vi "uLTV_main.vi"() -> ()   [LabVIEW 2021]
uses:
  <vilib>/myRIO/Instrument Drivers/Onboard IO/DIO/typedefs/DIO Reference.ctl
  <vilib>/myRIO/Common/Instrument Driver Framework/Utilities/typedefs/myRIO Generic Hardware Reference.ctl
  <vilib>/myRIO/Common/Instrument Driver Framework/Utilities/typedefs/Hardware Version Enum.ctl
  <vilib>/myRIO/Common/Instrument Driver Framework/Utilities/typedefs/myRIO v1.0 Reference.ctl
  <vilib>/myRIO/Common/Instrument Driver Framework/Utilities/typedefs/Generic FPGA Reference.ctl
  <vilib>/myRIO/Common/Instrument Driver Framework/myRIO v1.0/DIO/typedefs/DIO Channels List.ctl
  <vilib>/myRIO/Common/Instrument Driver Framework/myRIO v1.0/DIO/typedefs/DIO Channels Enum.ctl
  <vilib>/userDefined/High Color/nirio_resource_hc.ctl
  <vilib>/myRIO/Instrument Drivers/Onboard IO/PWM/typedefs/PWM Reference.ctl
  <vilib>/myRIO/Common/Instrument Driver Framework/myRIO v1.0/PWM/typedefs/PWM Channels Enum.ctl
  <vilib>/myRIO/Instrument Drivers/Onboard IO/PWM/typedefs/PWM Configuration.ctl
  <vilib>/myRIO/Common/Instrument Driver Framework/Utilities/vis/Is FPGA Ref Available.vi
  <vilib>/myRIO/Common/Instrument Driver Framework/myRIO v1.0/DIO/vis/myRIO v1.1 Open DIO.vi
  <vilib>/myRIO/Instrument Drivers/Onboard IO/DIO/vis/Write.vi
  <vilib>/myRIO/Common/Instrument Driver Framework/myRIO v1.0/PWM/vis/myRIO v1.1 Open PWM.vi
  <vilib>/myRIO/Instrument Drivers/Onboard IO/PWM/vis/Set Duty Cycle and Frequency.vi
  <vilib>/myRIO/Common/Instrument Driver Framework/Utilities/vis/Validate Channels.vi
  <vilib>/myRIO/Common/Instrument Driver Framework/myRIO v1.0/DIO/vis/myRIO v1.0 Reserve DIO.vi
  <vilib>/myRIO/Common/Instrument Driver Framework/myRIO v1.0/PWM/vis/myRIO v1.0 Reserve PWM.vi
  <vilib>/myRIO/Common/Instrument Driver Framework/myRIO v1.0/Resource Manager/vis/myRIO v1.0 Reserve Channel List.vi
  <vilib>/myRIO/Common/Instrument Driver Framework/myRIO v1.0/DIO/vis/myRIO v1.0 Build MUX Configuration DIO.vi
  <vilib>/myRIO/Common/Instrument Driver Framework/myRIO v1.0/PWM/vis/myRIO v1.0 Build MUX Configuration PWM.vi
  <vilib>/myRIO/Common/Instrument Driver Framework/myRIO v1.0/Resource Manager/vis/myRIO v1.0 Reserve Channel.vi
  <vilib>/myRIO/Common/Instrument Driver Framework/myRIO v1.0/Resource Manager/vis/myRIO v1.0 Unreserve Channel.vi
  <vilib>/myRIO/Common/Instrument Driver Framework/myRIO v1.0/Resource Manager/vis/myRIO v1.0 Create Configuration List.vi
  <vilib>/myRIO/Common/Instrument Driver Framework/myRIO v1.0/Resource Manager/vis/myRIO v1.0 Build Mutex Name.vi
  <vilib>/Utility/VariantDataType/GetNumericInfo.vi
  <vilib>/Utility/error.llb/Error Cluster From Error Code.vi
  <vilib>/myRIO/Common/Instrument Driver Framework/myRIO v1.0/myRIO v1.1 Open.vi
  <vilib>/myRIO/Common/Instrument Driver Framework/Utilities/vis/IO Manager.vi
  <vilib>/myRIO/Common/Instrument Driver Framework/Utilities/vis/Configuration Manager.vi
  <vilib>/myRIO/Common/Instrument Driver Framework/myRIO v1.0/Resource Manager/vis/myRIO v1.0 Configure IO.vi
  <vilib>/myRIO/Common/Instrument Driver Framework/myRIO v1.0/myRIO v1.0 Close.vi
  <vilib>/myRIO/Common/Instrument Driver Framework/myRIO v1.0/PWM/vis/myRIO v1.0 Write PWM.vi
  <vilib>/myRIO/Common/Instrument Driver Framework/myRIO v1.0/DIO/vis/myRIO v1.0 Write DIO.vi
  <vilib>/myRIO/Express VI/Onboard IO/PWM/PWM Express VI.xnode
  <vilib>/myRIO/Instrument Drivers/Onboard IO/PWM/vis/myRIO PWM Open.xnode
  <vilib>/myRIO/Express VI/Onboard IO/DO/DO Express VI.xnode
  <vilib>/myRIO/Instrument Drivers/Onboard IO/DIO/vis/myRIO DIO Open.xnode
  <vilib>/myRIO/Instrument Drivers/Onboard IO/PWM/PWM.lvlib
  <vilib>/myRIO/Instrument Drivers/Onboard IO/DIO/DIO.lvlib
panel:
  out "A/DIO0 (Pin 11) 4":bool
  out "A/DIO0 (Pin 11) 3":bool
  out "A/DIO0 (Pin 11) 2":bool
  out "A/DIO0 (Pin 11)":bool
  in  "Frequency [Hz]":dbl=1000.0
  out "Angle":dbl
  out "Magnitude":dbl
  in  "stop":bool
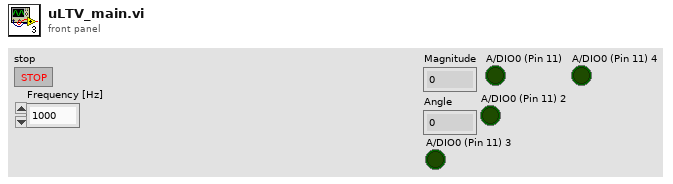
[diagram p1: front panel]
types:
  T1 = typedef "DIO.lvlib/DIO Reference.ctl" = cluster{"myRIO Reference":T2, "DIO Channels List":T6}
  T2 = typedef "myRIO Generic Hardware Reference.ctl" = cluster{"myRIO Model":T3, "myRIO Hardware Reference":T4}
  T3 = typedef "Hardware Version Enum.ctl" = enum16{"Unknown", "myRIO-1900", "myRIO-1950", "roboRIO", "NI ELVIS RIO CM", "ELVIS III"}
  T4 = typedef "myRIO v1.0 Reference.ctl" = cluster{"Generic FPGA Reference":T5, "Allow multiple opens":bool}
  T5 = typedef "Generic FPGA Reference.ctl" = refnum<k20>
  T6 = typedef "DIO Channels List.ctl" = T7[]
  T7 = typedef "DIO Channels Enum.ctl" = enum16{"Not Connected", "C/DIO0", "C/DIO1", "C/DIO2", "C/DIO3", "C/DIO4", "C/DIO5", "C/DIO6", "C/DIO7", "A/DIO0", "A/DIO1", "A/DIO2", "A/DIO3", "A/DIO4", "A/DIO5", "A/DIO6", "A/DIO7", "A/DIO8", "A/DIO9", "A/DIO10", "A/DIO11", "A/DIO12", "A/DIO13", "A/DIO14", "A/DIO15", "A/DIO16", "A/DIO17", "A/DIO18", "A/DIO19", "B/DIO0", "B/DIO1", "B/DIO2", "B/DIO3", "B/DIO4", "B/DIO5", "B/DIO6", "B/DIO7", "B/DIO8", "B/DIO9", "B/DIO10", "B/DIO11", "B/DIO12", "B/DIO13", "B/DIO14", "B/DIO15", "B/DIO16", "B/DIO17", "B/DIO18", "B/DIO19", "LED0", "LED1", "LED2", "LED3", "Button0", "DIO/DIO0", "DIO/DIO1", "DIO/DIO2", "DIO/DIO3", "DIO/DIO4", "DIO/DIO5", "DIO/DIO6", "DIO/DIO7", "DIO/DIO8", "DIO/DIO9", "SPI/CS0", "SPI/CS1", "SPI/CS2", "SPI/CS3", "LED RADIO (Green)", "LED RADIO (Red)", "LED COMM (Green)", "LED COMM (Red)", "LED MODE (Green)", "LED MODE (Red)"}
  T8 = typedef "nirio_resource_hc.ctl" = tag
  T9 = typedef "PWM.lvlib/PWM Reference.ctl" = cluster{"myRIO Reference":T2, "PWM Channels Enum":T10, "PWM Configuration":T11}
  T10 = typedef "PWM Channels Enum.ctl" = enum16{"Not Connected", "C/PWM0", "C/PWM1", "A/PWM0", "A/PWM1", "A/PWM2", "A/PWM3", "A/PWM4", "A/PWM5", "A/PWM6", "A/PWM7", "A/PWM8", "A/PWM9", "A/PWM10", "A/PWM11", "A/PWM12", "A/PWM13", "A/PWM14", "A/PWM15", "A/PWM16", "A/PWM17", "A/PWM18", "A/PWM19", "B/PWM0", "B/PWM1", "B/PWM2", "B/PWM3", "B/PWM4", "B/PWM5", "B/PWM6", "B/PWM7", "B/PWM8", "B/PWM9", "B/PWM10", "B/PWM11", "B/PWM12", "B/PWM13", "B/PWM14", "B/PWM15", "B/PWM16", "B/PWM17", "B/PWM18", "B/PWM19", "PWM/PWM0", "PWM/PWM1", "PWM/PWM2", "PWM/PWM3", "PWM/PWM4", "PWM/PWM5", "PWM/PWM6", "PWM/PWM7", "PWM/PWM8", "PWM/PWM9"}
  T11 = typedef "PWM.lvlib/PWM Configuration.ctl" = cluster{"Frequency":dbl, "Duty Cycle":dbl}
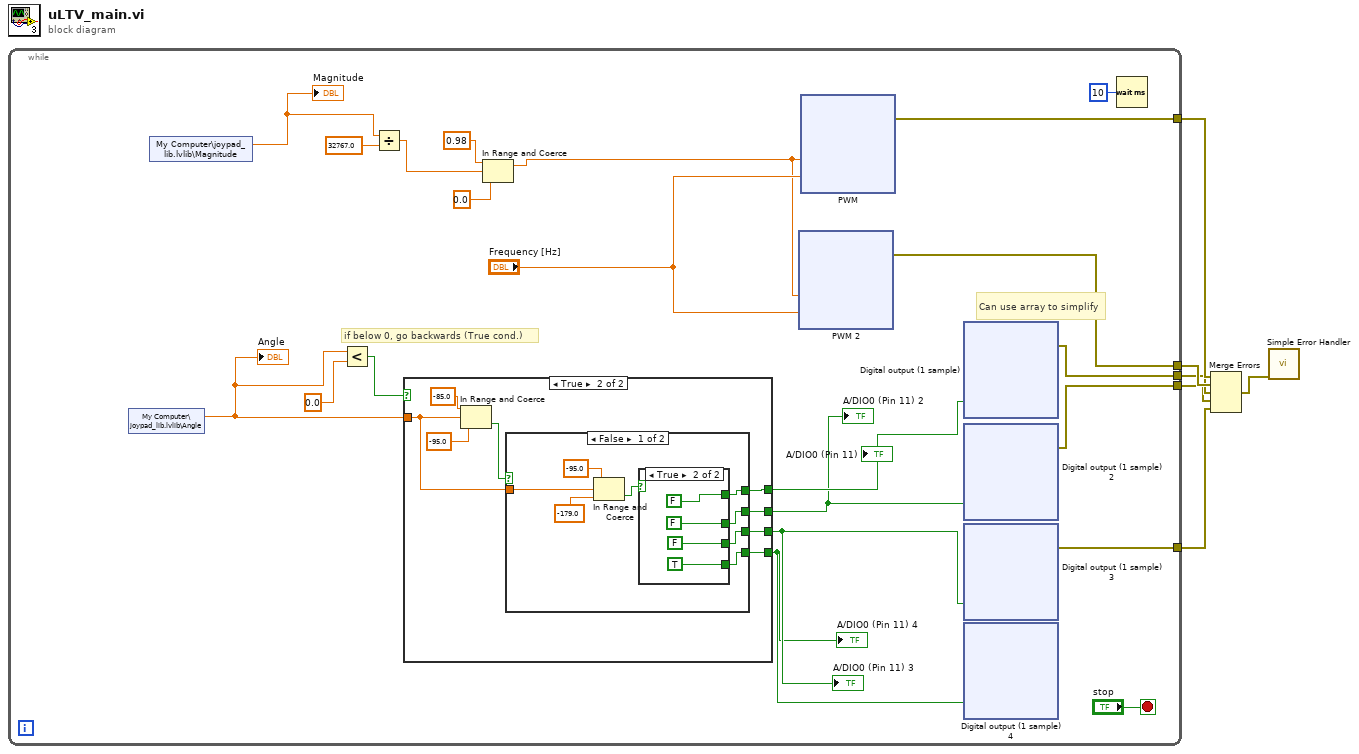
[diagram p0: block diagram]
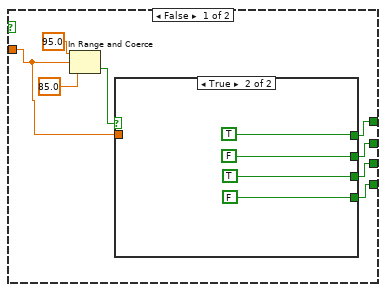
[diagram p2: hidden frame]
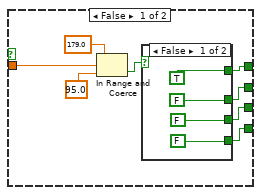
[diagram p3: hidden frame]
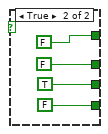
[diagram p4: hidden frame]
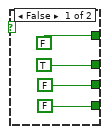
[diagram p5: hidden frame]
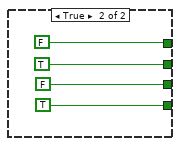
[diagram p6: hidden frame]
diagram:
  n1 = while {
    tunnel: [w17] -> w5
    tunnel: [w16] -> w4
    tunnel: [w15] -> w3
    tunnel: [w14] -> w2
    tunnel: [w13] -> w1
    stop <- "stop" stop-if-true
    # "Can use array to simplify"
    # "if below 0, go backwards (True cond.)"
    n2 = shared-variable "My Computer\\joypad_lib.lvlib\\Angle"() -> (w12:dbl)  [unwired: 1 in, 1 out]
    "Angle" <- w12
    n3 = shared-variable "My Computer\\joypad_lib.lvlib\\Magnitude"() -> (w22:dbl)  [unwired: 1 in, 1 out]
    "Magnitude" <- w22
    n4 = Less?(x=w12, y=0.0) -> (x < y?=w18:bool)
    n5 = Divide(x=w22, y=32767.0) -> (x/y=w21:dbl)
    n6 = case shown="True" w18 {
      tunnel: w12 -> [w172 w200]
      tunnel: [w171 w197] -> w11
      tunnel: [w170 w199] -> w9
      tunnel: [w169 w198] -> w8
      tunnel: [w168 w196] -> w7
      frame False {
        n7 = In Range and Coerce(upper limit=95.0, x=w172, lower limit=85.0) -> (In Range?=w173:bool)  [unwired: 1 out]
        n8 = case shown="True" w173 {
          tunnel: w172 -> [w181 _]
          tunnel: [w179 FALSE ("A/DIO0 (Pin 11)")] -> w170
          tunnel: [w178 TRUE ("A/DIO0 (Pin 11)")] -> w169
          tunnel: [w177 TRUE ("A/DIO0 (Pin 11)")] -> w171
          tunnel: [w176 FALSE ("A/DIO0 (Pin 11)")] -> w168
          frame False {
            n9 = In Range and Coerce(upper limit=179.0, x=w181, lower limit=95.0) -> (In Range?=w180:bool)  [unwired: 1 out]
            n10 = case shown="False" w180 {
              tunnel: [TRUE ("A/DIO0 (Pin 11)") FALSE ("A/DIO0 (Pin 11)")] -> w177
              tunnel: [FALSE ("A/DIO0 (Pin 11)") FALSE ("A/DIO0 (Pin 11)")] -> w179
              tunnel: [FALSE ("A/DIO0 (Pin 11)") TRUE ("A/DIO0 (Pin 11)")] -> w178
              tunnel: [FALSE ("A/DIO0 (Pin 11)") FALSE ("A/DIO0 (Pin 11)")] -> w176
              frame False {
              }
              frame True {
              }
            }
          }
          frame True {
          }
        }
      }
      frame True {
        n11 = In Range and Coerce(upper limit=-85.0, x=w200, lower limit=-95.0) -> (In Range?=w201:bool)  [unwired: 1 out]
        n12 = case shown="False" w201 {
          tunnel: w200 -> [w209 _]
          tunnel: [w207 TRUE ("A/DIO0 (Pin 11)")] -> w199
          tunnel: [w206 FALSE ("A/DIO0 (Pin 11)")] -> w198
          tunnel: [w205 FALSE ("A/DIO0 (Pin 11)")] -> w197
          tunnel: [w204 TRUE ("A/DIO0 (Pin 11)")] -> w196
          frame False {
            n13 = In Range and Coerce(upper limit=-95.0, x=w209, lower limit=-179.0) -> (In Range?=w208:bool)  [unwired: 1 out]
            n14 = case shown="True" w208 {
              tunnel: [FALSE ("A/DIO0 (Pin 11)") FALSE ("A/DIO0 (Pin 11)")] -> w205
              tunnel: [TRUE ("A/DIO0 (Pin 11)") FALSE ("A/DIO0 (Pin 11)")] -> w207
              tunnel: [FALSE ("A/DIO0 (Pin 11)") FALSE ("A/DIO0 (Pin 11)")] -> w206
              tunnel: [FALSE ("A/DIO0 (Pin 11)") TRUE ("A/DIO0 (Pin 11)")] -> w204
              frame False {
              }
              frame True {
              }
            }
          }
          frame True {
          }
        }
      }
    }
    "A/DIO0 (Pin 11)" <- w11
    "A/DIO0 (Pin 11) 2" <- w9
    "A/DIO0 (Pin 11) 3" <- w8
    "A/DIO0 (Pin 11) 4" <- w7
    n15 = In Range and Coerce(upper limit=0.98, x=w21, lower limit=0.0) -> (coerced(x)=w10:dbl)  [unwired: 1 out]
    n16 = xnode "PWM 2"("Duty Cycle"=w10, "Frequency [Hz]"="Frequency [Hz]") -> ("error out"=w16:errorcluster)  [unwired: 1 in]
    n17 = xnode "PWM"("Duty Cycle"=w10, "Frequency [Hz]"="Frequency [Hz]") -> ("error out"=w17:errorcluster)  [unwired: 1 in]
    n18 = xnode "Digital output (1 sample)"("A/DIO0 (Pin 11)"=w11) -> ("error out"=w15:errorcluster)  [unwired: 1 in]
    n19 = xnode "Digital output (1 sample) 2"("A/DIO1 (Pin 13)"=w9) -> ("error out"=w14:errorcluster)  [unwired: 1 in]
    n20 = xnode "Digital output (1 sample) 3"("A/DIO2 (Pin 15)"=w8) -> ("error out"=w13:errorcluster)  [unwired: 1 in]
    n21 = xnode "Digital output (1 sample) 4"("A/DIO3 (Pin 17)"=w7) -> ()  [unwired: 1 in, 1 out]
    n22 = Wait (ms)(milliseconds to wait=u32 10) -> ()  [unwired: 1 out]
  }
  n23 = Merge Errors(w5, w4, w3, w2, w1) -> (w6:errorcluster)
  n24 = call <vilib>:"Simple Error Handler.vi"("error in (no error)"=w6) -> ()  [unwired: 4 in, 5 out]
